vi "Init.vi"(8 "error in (no error)":errorcluster, 10 "Channel":i16, 11 "TrialBasedExperiment in":refnum<class "FleTraining.lvclass">) -> (0 "error out":errorcluster, 3 "TrialBasedExperiment out":refnum<class "FleTraining.lvclass">)   [LabVIEW 2012, in "FleTraining.lvclass"]
uses:
  FleTraining.lvclass
  TwoAfcEye/TwoAfcEye.lvclass
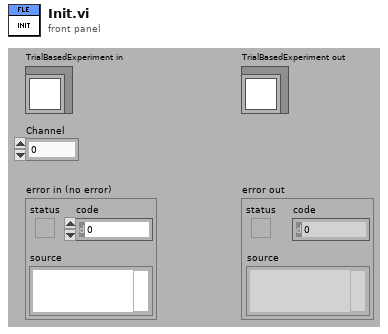
[diagram p1: front panel]
types:
  T1 = cluster{"Intertrial":dbl, "AcquireFixation":dbl, "HoldFixation":dbl, "DelayPeriod":dbl, "ResponsePeriod":dbl}
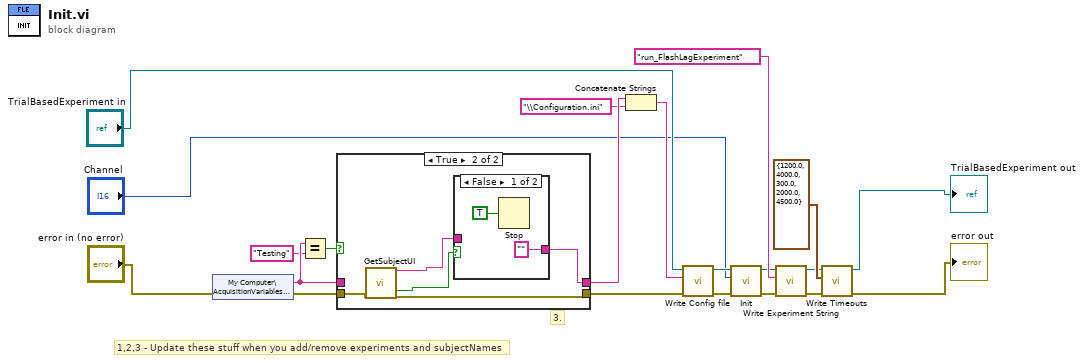
[diagram p0: block diagram]
diagram:
  # "1,2,3 - Update these stuff when you add/remove experiments and subjectNames"
  # "3."
  n1 = shared-variable "My Computer\\AcquisitionVariables.lvlib\\Subject"(error in="error in (no error)") -> (w12:string, error out=w13:errorcluster)
  n2 = Equal?(x=w12, y="Testing") -> (x = y?=w10:bool)
  n3 = case shown="True" w10 {
    tunnel: [w23 w28] -> w21
    tunnel: w12 -> [w23 _]
    tunnel: w13 -> [w22 w24]
    tunnel: [w22 w25] -> w14
    frame False {
    }
    frame True {
      n4 = call "GetSubjectUI.vi"("error in (no error)"=w24) -> ("subjectSelected"=w27:string, "OK"=w26:bool, "error out"=w25:errorcluster)  [unwired: 16 in]
      n5 = case shown="False" w26 {
        tunnel: w27 -> [_ w31]
        tunnel: ["" ("subjectSelected") w31] -> w28
        frame False {
          n6 = Stop(stop? (T)=TRUE) -> ()
        }
        frame True {
        }
      }
    }
  }
  n7 = Concatenate Strings(w21, "\\Configuration.ini") -> (w8:string)
  n8 = call-dynamic "Write Config file.vi"("error in (no error)"=w14, "Config file"=w8, "TrialBasedExperiment in"="TrialBasedExperiment in") -> ("error out"=w15:errorcluster, "TrialBasedExperiment out"=w16:refnum<class "FleTraining.lvclass">)  [unwired: 7 in]
  n9 = call-parent "Init.vi"("error in (no error)"=w15, "Channel"="Channel", "TrialBasedExperiment in"=w16) -> ("error out"=w18:errorcluster, "TrialBasedExperiment out"=w17:refnum<class "FleTraining.lvclass">)  [unwired: 7 in]
  n10 = call-dynamic "Write Experiment String.vi"("error in (no error)"=w18, "Experiment String"="run_FlashLagExperiment" ("string"), "TrialBasedExperiment in"=w17) -> ("error out"=w7:errorcluster, "TrialBasedExperiment out"=w6:refnum<class "FleTraining.lvclass">)  [unwired: 7 in]
  n11 = call-dynamic "Write Timeouts.vi"("error in (no error)"=w7, "Timeouts"=T1 {"Intertrial"=1200.0, "AcquireFixation"=4000.0, "HoldFixation"=300.0, "DelayPeriod"=2000.0, "ResponsePeriod"=4500.0}, "TrialBasedExperiment in"=w6) -> ("error out"=→"error out":errorcluster, "TrialBasedExperiment out"=→"TrialBasedExperiment out":refnum<class "FleTraining.lvclass">)  [unwired: 7 in]
